vi "KH_DAQ_TURCK_StatusDXP Write.vi"(11 "TBEN-S1-8DXP Input Values":T1) -> (3 "Status DXP":bool[](array[boolean]))   [LabVIEW 2021]
uses:
  KH Turck EthernetIP 17.12/KH TURCK ETHERNETIP TDefCluster TBEN-S1-8DXP Input Values.ctl
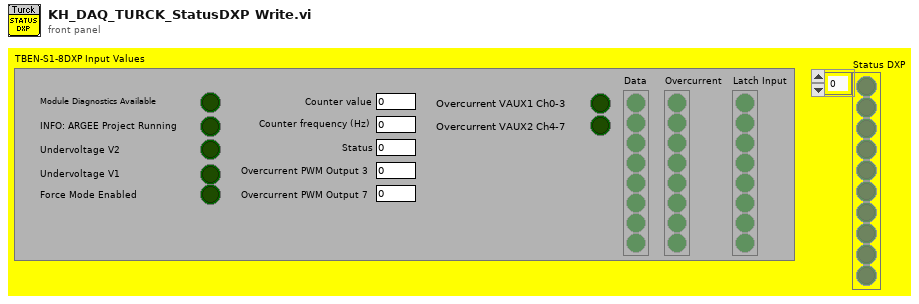
[diagram p1: front panel]
types:
  T1 = typedef "KH TURCK ETHERNETIP TDefCluster TBEN-S1-8DXP Input Values.ctl" = cluster{"Data":bool[], "Overcurrent":bool[], "Overcurrent VAUX1 Ch0-3":bool, "Overcurrent VAUX2 Ch4-7":bool, "Latch Input":bool[], "Counter value":u32, "Counter frequency (Hz)":u16, "Status":u8, "Overcurrent PWM Output 3":u8, "Overcurrent PWM Output 7":u8, "Module Diagnostics Available":bool, "INFO: ARGEE Project Running":bool, "Undervoltage V2":bool, "Undervoltage V1":bool, "Force Mode Enabled":bool}
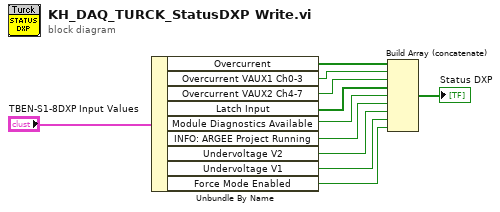
[diagram p0: block diagram]
diagram:
  n1 = Unbundle By Name("TBEN-S1-8DXP Input Values") -> ("Overcurrent"=w10:bool[], "Overcurrent VAUX1 Ch0-3"=w9:bool, "Overcurrent VAUX2 Ch4-7"=w8:bool, "Latch Input"=w7:bool[], "Module Diagnostics Available"=w6:bool, "INFO: ARGEE Project Running"=w5:bool, "Undervoltage V2"=w4:bool, "Undervoltage V1"=w3:bool, "Force Mode Enabled"=w2:bool)
  n2 = Build Array (concatenate)(w10, w9, w8, w7, w6, w5, w4, w3, w2) -> (→"Status DXP":bool[])
